vi "File.Find File in Folder using pattern.vi"(8 "error in (no error)":errorcluster, 10 "Pattern":string, 11 "Folder":path) -> (0 "error out":errorcluster, 2 "File Name":string, 3 "Found File":path)   [LabVIEW 2024]
uses:
  Errors/Error.Error Code List.ctl
  <vilib>/KATE/Files/File Utils.lvlib
  Errors.lvlib
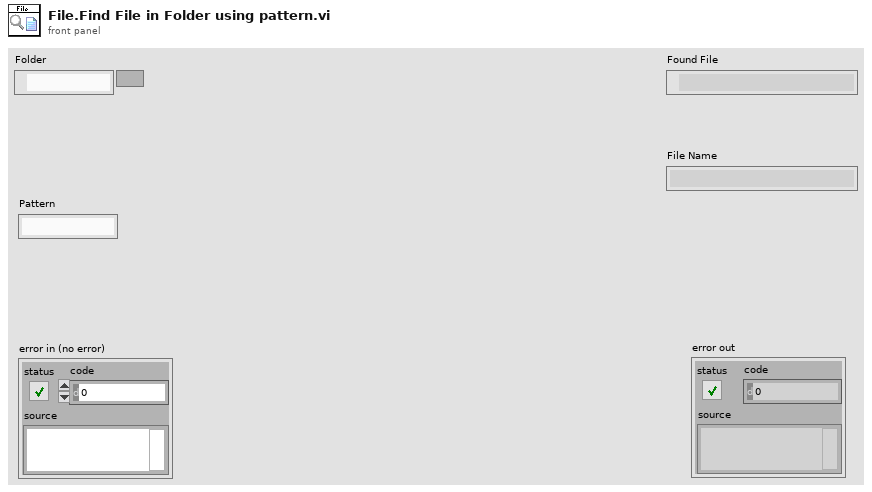
[diagram p1: front panel]
types:
  T1 = typedef "EQMF.lvlib/Errors.lvlib/Error.Error Code List.ctl" = i32
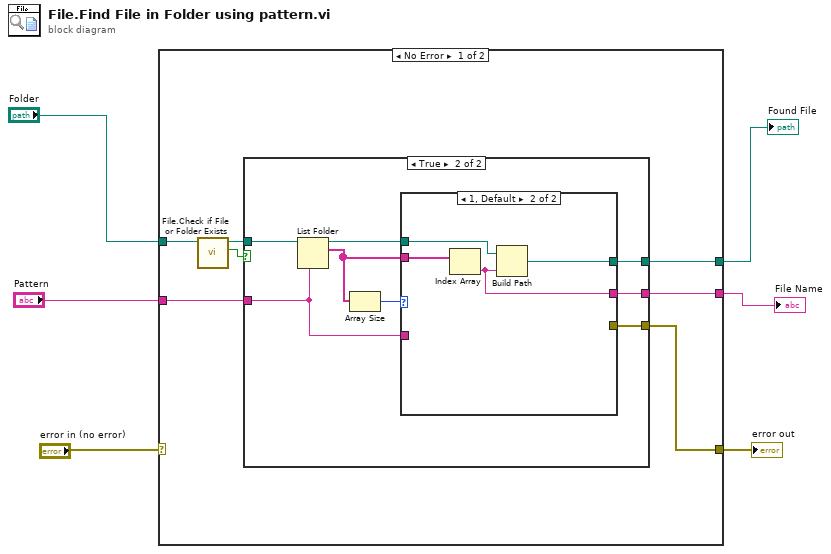
[diagram p0: block diagram]
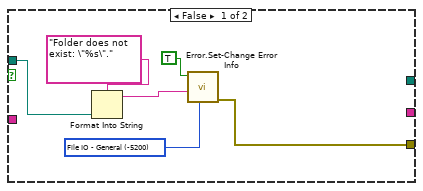
[diagram p2: hidden frame]
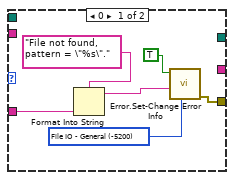
[diagram p3: hidden frame]
diagram:
  n1 = case shown="No Error" "error in (no error)" {
    selector: "error in (no error)" -> [_ w38]
    tunnel: "Folder" -> [w11 _]
    tunnel: [w13 _] -> w5
    tunnel: "Pattern" -> [w12 _]
    tunnel: [w8 w38] -> w2
    tunnel: [w7 _] -> w1
    frame No Error {
      n2 = call <vilib>:"File.Check if File or Folder Exists.vi"("Path"=w11) -> ("Exists"=w9:bool, "Dup Path"=w10:path)  [unwired: 6 in, 3 out]
      n3 = case shown="True" w9 {
        tunnel: [_ w26] -> w13
        tunnel: w12 -> [_ w22]
        tunnel: w10 -> [w15 w25]
        tunnel: [w18 w21] -> w8
        tunnel: [_ w20] -> w7
        frame False {
          w14 = T1 -5200 items=["No Error"=0, "Abort"=-2, "Misc"=-5000, "Fixture Error"=-5100, "File IO - General"=-5200, "FIle IO - Config Error"=-5201, "Instrument - General"=-5300, "Instrument - Serial Com"=-5301, "Instrument - Camera"=-5302, "Instrument - PS"=-5303, "Instrument - Oscilloscope"=-5304, "Instrument - Function Gen"=-5305, "Instrument - Load"=-5306, "Instrument - Meter"=-5307, "Instrument - Power Control"=-5308, "Instrument - Motion"=-5309, "Instrument - RF"=-5310, "System Exe"=-5400, "Image Processing"=-5500, "Communication"=-5600, "Script - Syntax Error"=-6000, "Script - Invalid Name or Param"=-6100, "Script - Timeout"=-6200, "Invalid Data"=-6300, "FW Update Error"=-6500] ("Std Code")
          n4 = Format Into String(format string="Folder does not exist: \"%s\"." ("Description"), w15) -> (resulting string=w16:string)  [unwired: 2 in, 1 out]
          n5 = call "Error.Set-Change Error Info.vi"("Std Code"=w14, "Description"=w16, "Set Error"=TRUE) -> ("error out"=w18:errorcluster)  [unwired: 8 in]
        }
        frame True {
          n6 = List Folder(path=w25, pattern=w22) -> (path out=w27:path, filenames=w24:string[])  [unwired: 2 in, 2 out]
          n7 = Array Size(array=w24) -> (size(s)=w23:i32)
          n8 = case shown="1, Default" w23 {
            tunnel: w27 -> [_ w37]
            tunnel: [_ w36] -> w26
            tunnel: w24 -> [_ w35]
            tunnel: w22 -> [w30 _]
            tunnel: [w28 _] -> w21
            tunnel: [_ w34] -> w20
            frame 0 {
              w29 = T1 -5200 items=["No Error"=0, "Abort"=-2, "Misc"=-5000, "Fixture Error"=-5100, "File IO - General"=-5200, "FIle IO - Config Error"=-5201, "Instrument - General"=-5300, "Instrument - Serial Com"=-5301, "Instrument - Camera"=-5302, "Instrument - PS"=-5303, "Instrument - Oscilloscope"=-5304, "Instrument - Function Gen"=-5305, "Instrument - Load"=-5306, "Instrument - Meter"=-5307, "Instrument - Power Control"=-5308, "Instrument - Motion"=-5309, "Instrument - RF"=-5310, "System Exe"=-5400, "Image Processing"=-5500, "Communication"=-5600, "Script - Syntax Error"=-6000, "Script - Invalid Name or Param"=-6100, "Script - Timeout"=-6200, "Invalid Data"=-6300, "FW Update Error"=-6500] ("Std Code")
              n9 = Format Into String(format string="File not found, pattern = \"%s\"." ("Description"), w30) -> (resulting string=w33:string)  [unwired: 2 in, 1 out]
              n10 = call "Error.Set-Change Error Info.vi"("Std Code"=w29, "Description"=w33, "Set Error"=TRUE) -> ("error out"=w28:errorcluster)  [unwired: 8 in]
            }
            frame 1, Default {
              n11 = Index Array(array=w35) -> (element=w34:string)  [unwired: 1 in]
              n12 = Build Path(base path=w37, name or relative path=w34) -> (appended path=w36:path)
            }
          }
        }
      }
    }
    frame Error {
    }
  }
  "Found File" <- w5
  "error out" <- w2
  "File Name" <- w1
